vi "GetCheckNo.vi"(1 "年月日":string="20181031", 2 "序号":u16=10, 4 "机台编号":string="FP-2871") -> (0 "CheckNo":string)   [LabVIEW 2018]
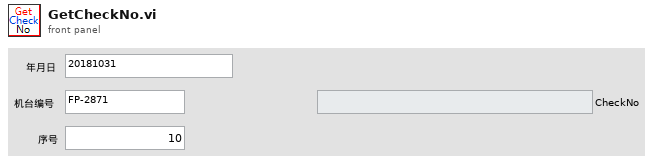
[diagram p1: front panel]
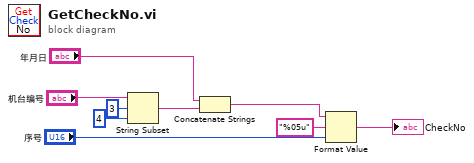
[diagram p0: block diagram]
diagram:
  n1 = String Subset(string="机台编号", offset (0)=3 ("偏移量(0)"), length (rest)=4 ("长度（剩余）")) -> (substring=w4:string)
  n2 = Concatenate Strings("年月日", w4) -> (w2:string)
  n3 = Format Value(string ("")=w2, format string="%05u" ("格式字符串"), value (0)="序号") -> (output string=→"CheckNo":string)
